vi "COMI US Cancel File Convert.vi"   [LabVIEW 2017, in "Comidll.lvlib"]
doc: "void (COMI_US_CancelFileConvert) (void);"
uses:
  <userlib>/Comidll/Comidll.lvlib
  <userlib>/Comidll/Comidll.dll
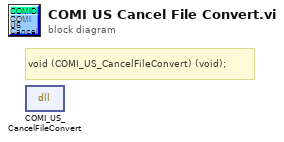
[diagram p0: block diagram]
diagram:
  # "void\t(COMI_US_CancelFileConvert) (void);"
  n1 = dll-call lib="C:/Program Files/National Instruments/LabVIEW 2017/user.lib/Comidll/Comidll.*" fn="COMI_US_CancelFileConvert"() -> ()  [unwired: 4 in, 2 out]
